vi "calc_displ_intens.vi"(9 "Avg intensity":T2(array[cluster]), 11 "Number of positions":i32) -> (2 "Intensity plot":T1)   [LabVIEW 2018]
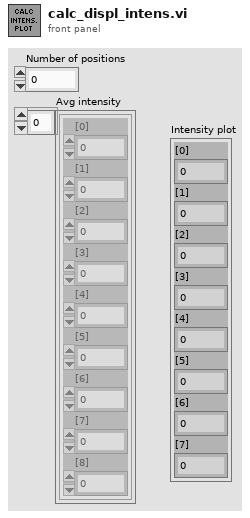
[diagram p1: front panel]
types:
  T1 = cluster{"[0]":dbl, "[1]":dbl, "[2]":dbl, "[3]":dbl, "[4]":dbl, "[5]":dbl, "[6]":dbl, "[7]":dbl}
  T2 = cluster{"[0]":dbl, "[1]":dbl, "[2]":dbl, "[3]":dbl, "[4]":dbl, "[5]":dbl, "[6]":dbl, "[7]":dbl, "[8]":dbl}[]
  T3 = cluster{"[0]":dbl, "[1]":dbl, "[2]":dbl, "[3]":dbl, "[4]":dbl, "[5]":dbl, "[6]":dbl, "[7]":dbl, "[8]":dbl}
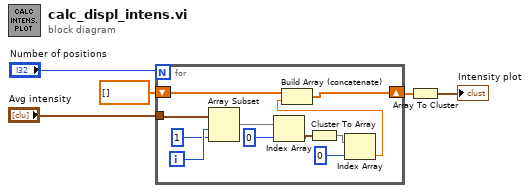
[diagram p0: block diagram]
diagram:
  n1 = for {
    N: "Number of positions" -> [_]
    shift-right: [w13] -> w4
    shift-left: dbl[] [] -> [w12]
    tunnel: "Avg intensity" -> [w14]
    i -> [w16]
    n2 = Array Subset(array=w14, index=w16, length=1) -> (w11:T2)
    n3 = Index Array(array=w11, index=0) -> (element=w9:T3)
    n4 = Cluster To Array(cluster=w9) -> (array=w7:dbl[])
    n5 = Index Array(array=w7, index=0) -> (element=w6:dbl)
    n6 = Build Array (concatenate)(w12, w6) -> (w13:dbl[])
  }
  n7 = Array To Cluster(array=w4) -> (cluster=→"Intensity plot":T1)
